vi "LED Graph.vi"() -> ()   [LabVIEW 2020, in "CTI-Scratchpad.lvlib"]
uses:
  CTI-Scratchpad.lvlib
  CTI/GPIO Number.ctl
  CTI/GPIO Direction.ctl
  CTI/Session/Session.lvclass
  CTI/CTI.lvlib
  CTI/VisaComms/VisaComms.lvclass
panel:
  out "Readback":bool[](array[boolean])
  in  "Port":refnum<visa-resource-name>="COM3"
  in  "stop":bool
  in  "Graph":u8(slide) scale=0.0..10.0
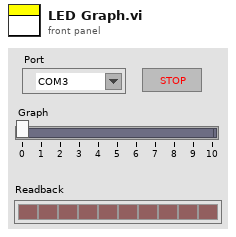
[diagram p1: front panel]
types:
  T1 = typedef "CTI.lvlib/GPIO Number.ctl" = i8
  T2 = typedef "CTI.lvlib/GPIO Direction.ctl" = enum16{"In", "Out"}
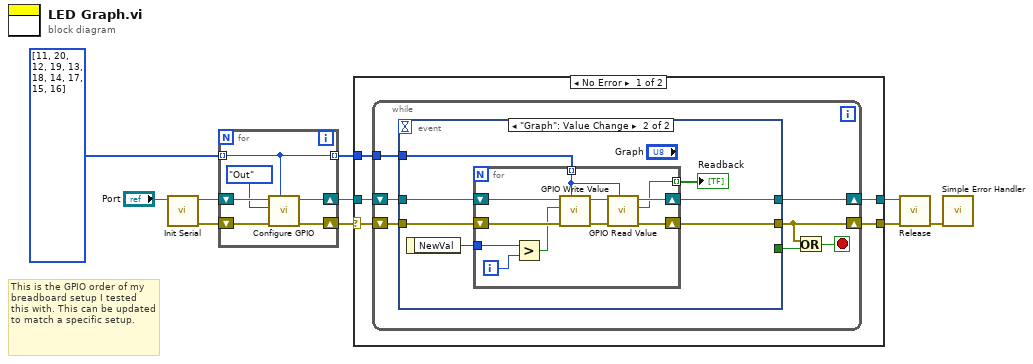
[diagram p0: block diagram]
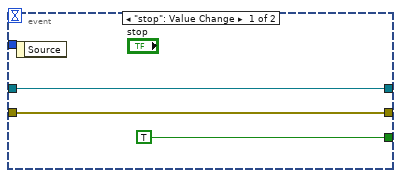
[diagram p2: hidden frame]
diagram:
  # "This is the GPIO order of my breadboard setup I tested this with. This can be updated to match a specific setup."
  n1 = call "Init Serial.vi"("VISA resource name in"="Port") -> ("error out"=w8:errorcluster, "Session"=w9:refnum<class "Session.lvclass">)  [unwired: 8 in, 1 out]
  n2 = for {
    tunnel: T1[] [11, 20, 12, 19, 13, 18, 14, 17, 15, 16] -> [w11] mode=indexing
    shift-right: [w14] -> w6
    shift-left: w8 -> [w15]
    shift-right: [w13] -> w7
    shift-left: w9 -> [w16]
    tunnel: [w11] -> w4 mode=indexing
    n3 = call "Configure GPIO.vi"("GPIO #"=w11, "error in (no error)"=w15, "GPIO Direction"=GPIO_Direction."Out", "Session in"=w16) -> ("error out"=w14:errorcluster, "Session out"=w13:refnum<class "Session.lvclass">)  [unwired: 6 in]
  }
  n4 = case shown="No Error" w6 {
    selector: w6 -> [w20 w50]
    tunnel: w7 -> [w21 w51]
    tunnel: w4 -> [w19 _]
    tunnel: [w18 w51] -> w2
    tunnel: [w17 w50] -> w3
    frame No Error {
      n5 = while {
        shift-right: [w26] -> w18
        shift-left: w21 -> [w28]
        shift-right: [w25] -> w17
        shift-left: w20 -> [w27]
        tunnel: w19 -> [w22]
        stop <- w24 stop-if-true
        n6 = event shown="[1] \"Graph\": Value Change" {
          selector: _ -> [_ _]
          dyn-events: _ -> [_ _]
          timeout: _ -> [_ _]
          tunnel: w28 -> [w31 w37]
          tunnel: w27 -> [w30 w36]
          tunnel: [w31 w34] -> w26
          tunnel: [w30 w33] -> w25
          tunnel: [TRUE _] -> w23
          tunnel: w22 -> [_ w35]
          event "stop": Value Change {
            n7 = event-data() -> ()  [unwired: 1 in, 1 out]
          }
          event "Graph": Value Change {
            n8 = event-data() -> ("NewVal"=w38:u8)  [unwired: 1 in]
            n9 = for {
              tunnel: w38 -> [w47]
              shift-right: [w43] -> w34
              shift-left: w37 -> [w49]
              shift-right: [w42] -> w33
              shift-left: w36 -> [w48]
              tunnel: w35 -> [w40] mode=indexing
              tunnel: [w41] -> w32 mode=indexing
              i -> [w46]
              n10 = Greater?(x=w47, y=w46) -> (0:w39:bool)
              n11 = call "GPIO Write Value.vi"("GPIO #"=w40, "error in (no error)"=w48, "Value"=w39, "Session in"=w49) -> ("error out"=w44:errorcluster, "Session out"=w45:refnum<class "Session.lvclass">)  [unwired: 6 in]
              n12 = call "GPIO Read Value.vi"("GPIO #"=w40, "error in (no error)"=w44, "Session in"=w45) -> ("error out"=w42:errorcluster, "Value"=w41:bool, "Session out"=w43:refnum<class "Session.lvclass">)  [unwired: 6 in]
            }
            "Readback" <- w32
          }
        }
        n13 = Or(x=w25, y=w23) -> (x .or. y?=w24:bool)
      }
    }
    frame Error {
    }
  }
  n14 = call-dynamic "Release.vi"("error in (no error)"=w3, "Session in"=w2) -> ("error out"=w1:errorcluster)  [unwired: 9 in]
  n15 = call <vilib>:"Simple Error Handler.vi"("error in (no error)"=w1) -> ()  [unwired: 4 in, 5 out]
